vi "Event Loop.vi"(8 "error in (no error)":errorcluster, 11 "Dynamic Combobox in":refnum<class "Dynamic Combobox.lvclass">) -> (0 "error out":errorcluster)   [LabVIEW 2020, in "Dynamic Combobox.lvlib" / "Dynamic Combobox.lvclass"]
uses:
  Dynamic Combobox.lvclass
  Loop State.ctl
  Dynamic Combobox.lvclass/Dynamic Combobox.ctl
  Incoming Events.ctl
panel:
  # "This is the Event Loop VI. This VI will be displayed when run when Debug is set to true with Init.vi"
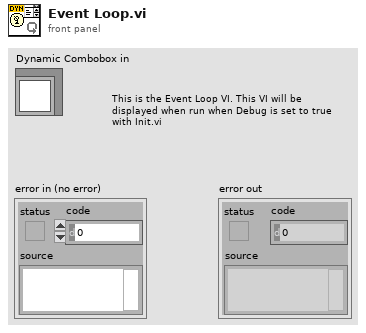
[diagram p1: front panel]
types:
  T1 = typedef "Dynamic Combobox.lvlib/Dynamic Combobox.lvclass/Loop State.ctl" = enum16{"Init", "Run", "Close"}
  T2 = enum8{"Enabled", "Disabled", "Disabled and Grayed Out"}
  T3 = enum32{"Invalid", "Standard", "Closed", "Hidden", "Minimized", "Maximized"}
  T4 = typedef "Dynamic Combobox.lvlib/Dynamic Combobox.lvclass/Incoming Events.ctl" = cluster{"Close":refnum<user-event>, "Refresh":refnum<user-event>}
  T5 = typedef "Dynamic Combobox.lvlib/Dynamic Combobox.lvclass/Ref Data.ctl" = cluster{"Values":refnum<class "Dynamic Values.lvclass">, "Debug":bool, "Strings And Values []":T6, "Options":T7}
  T6 = typedef "LVComboBoxStrsAndValuesArrayTypeDef.ctl" = cluster{"String":string, "Value":string}[]
  T7 = typedef "Dynamic Combobox.lvlib/Dynamic Combobox.lvclass/Options.ctl" = cluster{"Browse Entry":bool, "Refresh Entry":bool}
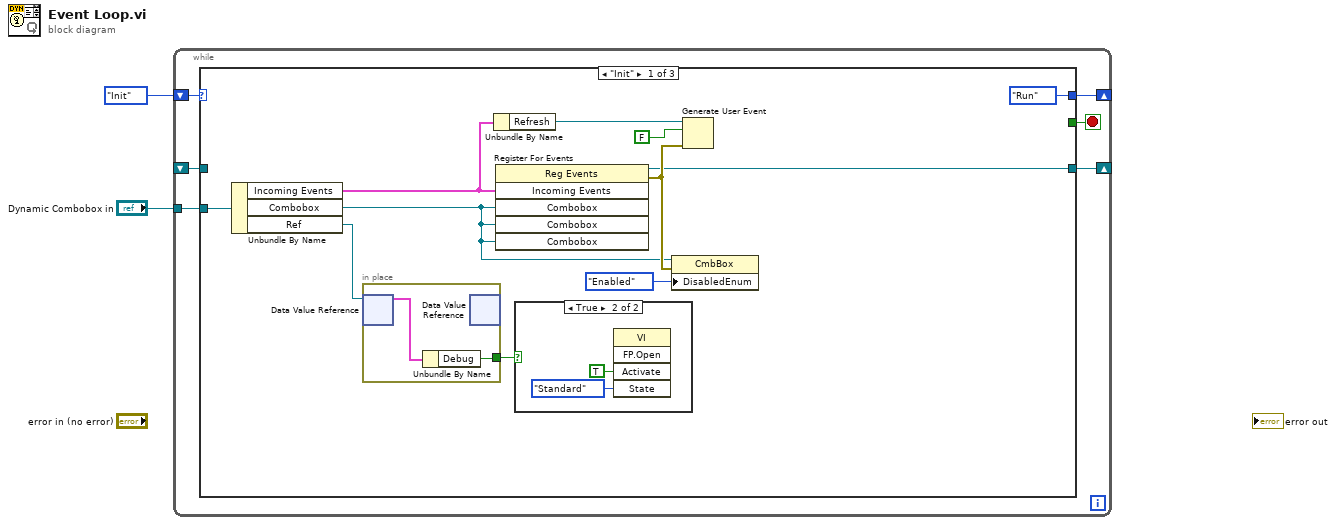
[diagram p0: block diagram]
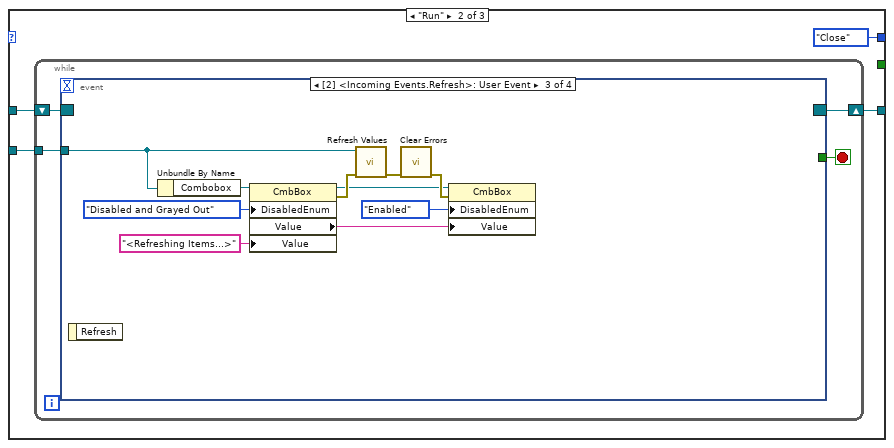
[diagram p3: hidden frame]
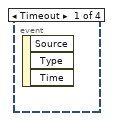
[diagram p4: hidden frame]
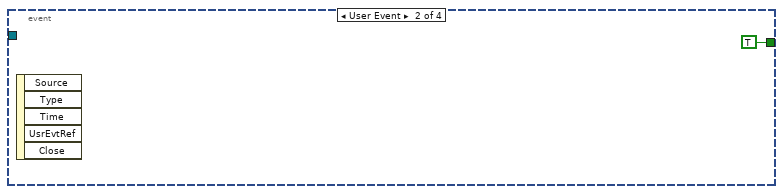
[diagram p5: hidden frame]
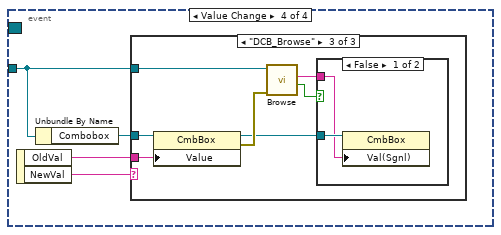
[diagram p6: hidden frame]
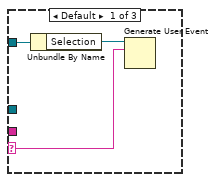
[diagram p7: hidden frame]
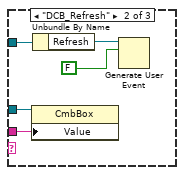
[diagram p8: hidden frame]
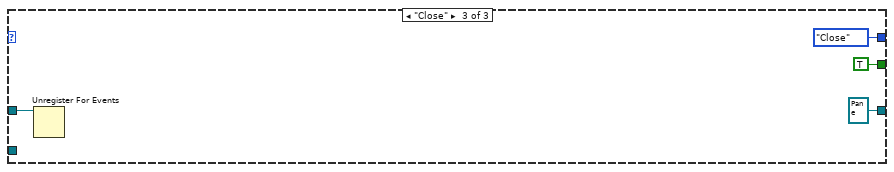
[diagram p10: hidden frame]
diagram:
  n1 = while {
    tunnel: "Dynamic Combobox in" -> [w8]
    shift-right: [w6] -> _
    shift-left: Loop_State."Init" ("Loop State") -> [w7]
    shift-right: [w4] -> _
    shift-left: _ -> [w3]
    stop <- w5 stop-if-true
    n2 = case shown="\"Init\"" w7 {
      tunnel: w8 -> [w18 w26 _]
      tunnel: [Loop_State."Run" ("Loop State") Loop_State."Close" ("Loop State") Loop_State."Close" ("Loop State")] -> w6
      tunnel: [_ _ TRUE] -> w5
      tunnel: [w13 w24 refnum<event-registration> refnum ("Event Registration Refnum")] -> w4
      tunnel: w3 -> [_ w25 w65]
      frame "Init" {
        n3 = Unbundle By Name(w18) -> ("Incoming Events"=w11:T4, "Combobox"=w14:refnum<vi>, "Ref"=w16:refnum<data-value>)
        n4 = in-place {
          in-place-border: [w22] -> w12
          n5 = in-place-dvr #1(w16) -> (w23:T5)  [unwired: 1 out]
          n6 = Unbundle By Name(w23) -> ("Debug"=w22:bool)
          n7 = in-place-dvr #1() -> ()  [unwired: 1 in, 2 out]
        }
        n8 = Unbundle By Name(w11) -> ("Refresh"=w10:refnum<user-event>)
        n9 = register-events(w11, w14, w14, w14) -> (reference out=w13:refnum<event-registration>, error out=w19:errorcluster)  [unwired: 2 in]
        n10 = case shown="True" w12 {
          frame False {
          }
          frame True {
            n11 = invoke class="VI" method="FP.Open"("Activate"=TRUE ("Activate?"), "State"=T3."Standard") -> ()  [unwired: 3 in, 5 out]
          }
        }
        n12 = property class="CmbBox"(reference=w14, error in=w19, "DisabledEnum"=T2."Enabled" ("Disabled")) -> ()  [unwired: 2 out]
        n13 = Generate User Event(user event=w10, event data cluster=FALSE ("event data"), error in=w19) -> ()  [unwired: 1 in, 2 out]
      }
      frame "Run" {
        n14 = while {
          tunnel: w26 -> [w28]
          shift-right: [w30] -> w24
          shift-left: w25 -> [w31]
          stop <- w29 stop-if-true
          n15 = event shown="[2] <Incoming Events.Refresh>: User Event" {
            selector: w31 -> [_ _ _ _]
            dyn-events: [_ _ _ _] -> w30
            timeout: _ -> [_ _ _ _]
            tunnel: [_ TRUE _ _] -> w29
            tunnel: w28 -> [_ _ w36 w43]
            event Timeout {
              n16 = event-data() -> ()  [unwired: 1 in, 3 out]
            }
            event User Event {
              n17 = event-data() -> ()  [unwired: 1 in, 5 out]
            }
            event User Event {
              n18 = event-data() -> ()  [unwired: 1 in, 1 out]
              n19 = Unbundle By Name(w36) -> ("Combobox"=w35:refnum<vi>)
              n20 = property class="CmbBox"(reference=w35, "DisabledEnum"=T2."Disabled and Grayed Out" ("Disabled"), "Value"="<Refreshing Items...>") -> (reference out=w38:refnum<vi>, error out=w40:errorcluster, "Value"=w33:string)  [unwired: 1 in]
              n21 = call "Refresh Values.vi"("error in (no error)"=w40, "Dynamic Combobox in"=w36) -> ("error out"=w41:errorcluster)  [unwired: 8 in, 1 out]
              n22 = call <vilib>:"Clear Errors.vi"("error in (no error)"=w41) -> ("error out"=w42:errorcluster)  [unwired: 5 in, 1 out]
              n23 = property class="CmbBox"(reference=w38, error in=w42, "DisabledEnum"=T2."Enabled" ("Disabled"), "Value"=w33) -> ()  [unwired: 2 out]
            }
            event Value Change {
              n24 = event-data() -> ("OldVal"=w45:string, "NewVal"=w46:string)  [unwired: 1 in]
              n25 = Unbundle By Name(w43) -> ("Combobox"=w44:refnum<vi>)
              n26 = case shown="\"DCB_Browse\"" w46 {
                selector: w46 -> [w48 _ _]
                tunnel: w45 -> [_ w54 w56]
                tunnel: w44 -> [_ w53 w57]
                tunnel: w43 -> [w47 w52 w55]
                frame Default {
                  n27 = Unbundle By Name(w47) -> ("Selection"=w49:refnum<user-event>)
                  n28 = Generate User Event(user event=w49, event data cluster=w48) -> ()  [unwired: 2 in, 2 out]
                }
                frame "DCB_Refresh" {
                  n29 = property class="CmbBox"(reference=w53, "Value"=w54) -> ()  [unwired: 1 in, 2 out]
                  n30 = Unbundle By Name(w52) -> ("Refresh"=w51:refnum<user-event>)
                  n31 = Generate User Event(user event=w51, event data cluster=FALSE ("event data")) -> ()  [unwired: 2 in, 2 out]
                }
                frame "DCB_Browse" {
                  n32 = property class="CmbBox"(reference=w57, "Value"=w56) -> (reference out=w58:refnum<vi>, error out=w61:errorcluster)  [unwired: 1 in]
                  n33 = call "Browse.vi"("error in (no error)"=w61, "Dynamic Combobox in"=w55) -> ("Cancelled?"=w60:bool, "Selected Value"=w59:string)  [unwired: 6 in, 2 out]
                  n34 = case shown="False" w60 {
                    tunnel: w59 -> [w62 _]
                    tunnel: w58 -> [w63 _]
                    frame False {
                      n35 = property class="CmbBox"(reference=w63, "Val(Sgnl)"=w62) -> ()  [unwired: 1 in, 2 out]
                    }
                    frame True {
                      # "Cancelled or error. Errors are already sent in Browse.vi"
                    }
                  }
                }
              }
            }
          }
        }
      }
      frame "Close" {
        n36 = Unregister For Events(event registration refnum=w65) -> ()  [unwired: 1 in, 1 out]
      }
    }
  }
